vi "newTestStandLimitStep.vi"(0 "Engine Reference":refnum<k7>, 1 "High Limit":dbl, 2 "Low Limit":dbl=215.0, 3 "Precondition":string, 5 "Sequence File Ref":refnum<k7>, 7 "Step Name":string="num limit test", 9 "Requirement":string, 11 "error in":errorcluster, 12 "index":i32, 13 "Comparison Type":string="LT") -> (4 "Engine reference(out)":refnum<k7>, 6 "Sequence File Ref(out)":refnum<k7>, 15 "error out":errorcluster)   [LabVIEW 2009]
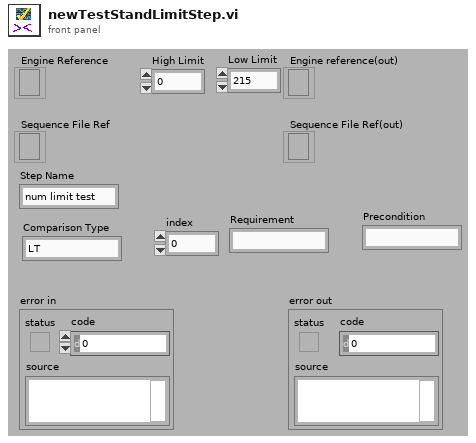
[diagram p1: front panel]
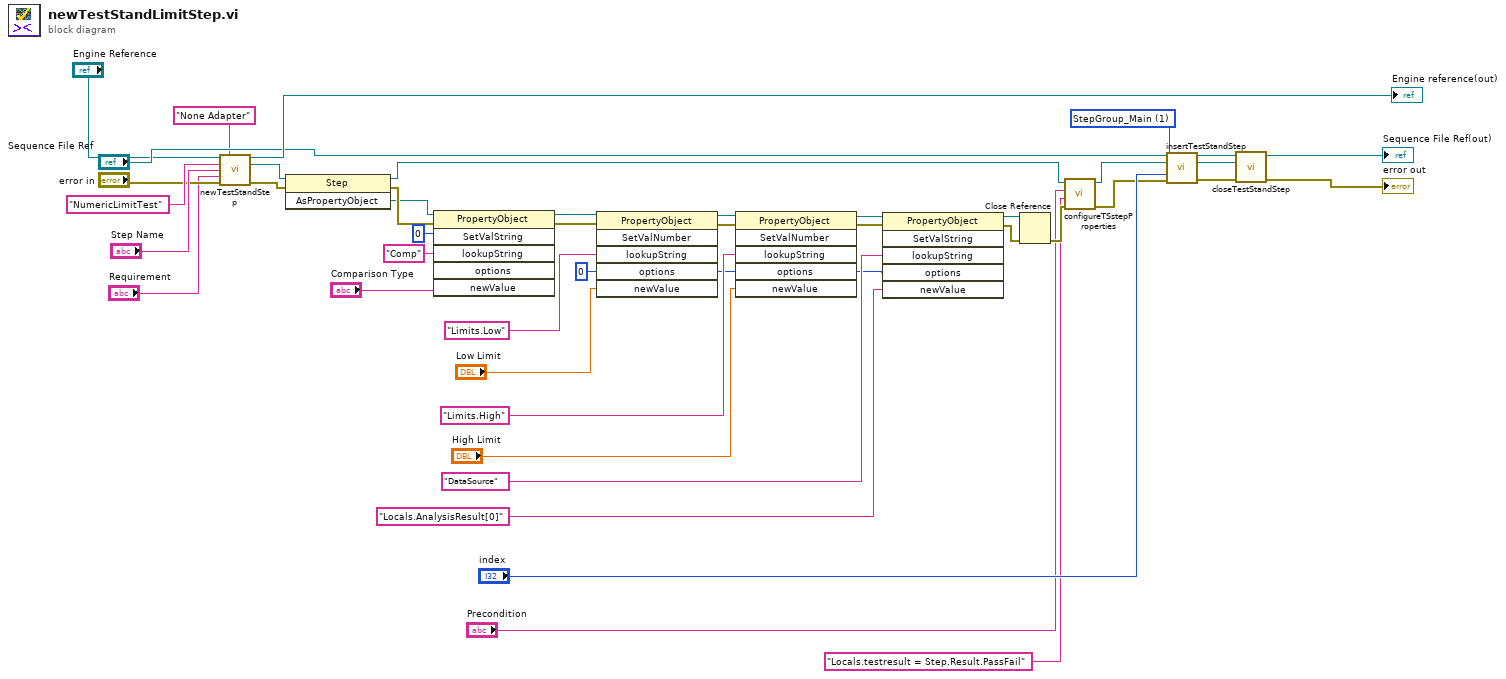
[diagram p0: block diagram]
diagram:
  w8 = 0 ("options")
  w26 = 1 items=["StepGroup_Setup", "StepGroup_Main", "StepGroup_Cleanup"] ("Step Group")
  n1 = call "newTestStandStep.vi"("Engine reference"="Engine Reference", "adapterKeyNameVal"="None Adapter", "stepType"="NumericLimitTest", "Step Name"="Step Name", "Requirement"="Requirement", "error in"="error in") -> ("Engine reference(out)"=→"Engine reference(out)":refnum<k7>, "NewStep (out)"=w33:refnum<k7>, "error out"=w34:errorcluster)  [unwired: 7 in]
  n2 = invoke class="Step" method="AsPropertyObject"(reference=w33, error in=w34) -> (reference out=w4:refnum<k7>, error out=w36:errorcluster, "AsPropertyObject"=w35:refnum<k7>)  [unwired: 1 in]
  n3 = invoke class="PropertyObject" method="SetValString"(reference=w35, error in=w36, "lookupString"="Comp", "options"=0, "newValue"="Comparison Type") -> (reference out=w40:refnum<k7>, error out=w41:errorcluster)  [unwired: 1 in, 4 out]
  n4 = invoke class="PropertyObject" method="SetValNumber"(reference=w40, error in=w41, "lookupString"="Limits.Low", "options"=w8, "newValue"="Low Limit") -> (reference out=w19:refnum<k7>, error out=w18:errorcluster)  [unwired: 1 in, 4 out]
  n5 = invoke class="PropertyObject" method="SetValNumber"(reference=w19, error in=w18, "lookupString"="Limits.High", "options"=w8, "newValue"="High Limit") -> (reference out=w13:refnum<k7>, error out=w12:errorcluster)  [unwired: 1 in, 4 out]
  n6 = invoke class="PropertyObject" method="SetValString"(reference=w13, error in=w12, "lookupString"="DataSource", "options"=w8, "newValue"="Locals.AnalysisResult[0]") -> (reference out=w11:refnum<k7>, error out=w10:errorcluster)  [unwired: 1 in, 4 out]
  n7 = Close Reference(reference=w11, error in (no error)=w10) -> (error out=w6:errorcluster)
  n8 = call "configureTSstepProperties.vi"("error in"=w6, "PostExpression"="Locals.testresult = Step.Result.PassFail", "Precondition"="Precondition", "NewStep (in)"=w4) -> ("error out"=w5:errorcluster, "NewStep (out)"=w3:refnum<k7>)  [unwired: 6 in]
  n9 = call "insertTestStandStep.vi"("Sequence File Ref"="Sequence File Ref", "Step to insert"=w3, "Step Group"=w26, "index"="index", "error out"=w5) -> ("Sequence File Ref(out)"=w29:refnum<k7>, "Step to insert (out)"=w28:refnum<k7>, "error out"=w27:errorcluster)  [unwired: 8 in]
  n10 = call "closeTestStandStep.vi"("error in"=w27, "NewStep"=w28, "Sequence File Ref"=w29) -> ("error out"=→"error out":errorcluster, "Sequence File Ref(out)"=→"Sequence File Ref(out)":refnum<k7>)  [unwired: 7 in]
